vi "IMAQ FPGA Camera Link Overflow Check.vi"(9 "Max Index":u16, 10 "Read Info":T2, 11 "Write Info":T3) -> (3 "Overlfow":bool)   [LabVIEW 2017]
uses:
  <vilib>/visionFPGA/Basics/Camera Link Acquisition/Controls/IMAQ FPGA Camera Link Line Builder State.ctl
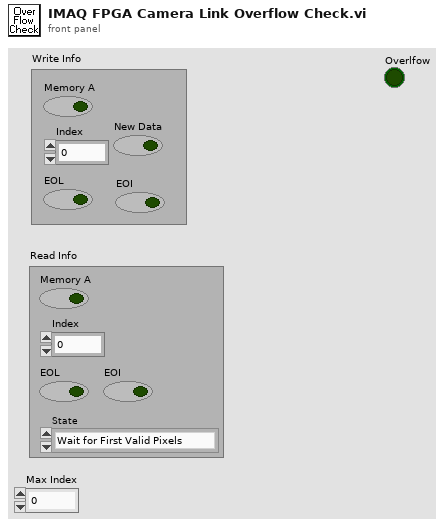
[diagram p1: front panel]
types:
  T1 = typedef "IMAQ FPGA Camera Link Line Builder State.ctl" = enum16{"Wait for First Valid Pixels", "Update Section 1", "Update Section 2", "Update Section 3", "Update Last Section", "Add Final Pack", "Add End of Line", "Check End of Image"}
  T2 = cluster{"Memory A":bool, "Index":u16, "EOL":bool, "State":T1, "EOI":bool}
  T3 = cluster{"Memory A":bool, "Index":u16, "EOL":bool, "New Data":bool, "EOI":bool}
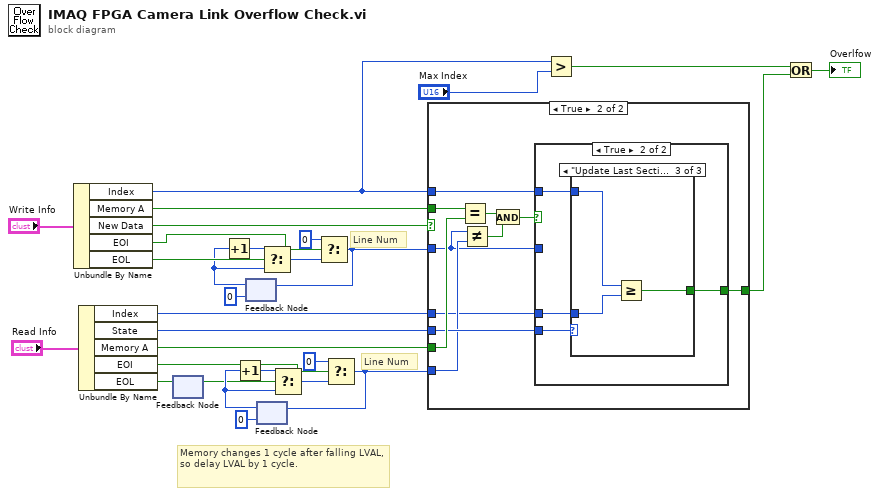
[diagram p0: block diagram]
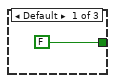
[diagram p4: hidden frame]
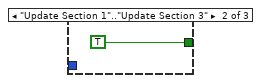
[diagram p5: hidden frame]
diagram:
  # "Line Num"
  # "Line Num"
  # "Memory changes 1 cycle after falling LVAL, so delay LVAL by 1 cycle."
  n1 = Unbundle By Name("Write Info") -> ("Index"=w7:u16, "Memory A"=w12:bool, "New Data"=w20:bool, "EOI"=w24:bool, "EOL"=w28:bool)
  n2 = Unbundle By Name("Read Info") -> ("Index"=w9:u16, "State"=w10:T1, "Memory A"=w11:bool, "EOI"=w13:bool, "EOL"=w14:bool)
  n3 = feedback-in #1(w14) -> ()
  n4 = feedback #1() -> (w8:bool)  [unwired: 1 in]
  n5 = feedback #2(u16 0) -> (w25:u16)
  n6 = Increment(x=w25) -> (x+1=w26:u16)
  n7 = feedback #3(u16 0) -> (w17:u16)
  n8 = Increment(x=w17) -> (x+1=w16:u16)
  n9 = Select(t=w26, s=w28, f=w25) -> (s? t:f=w23:u16)
  n10 = Select(t=w16, s=w8, f=w17) -> (s? t:f=w18:u16)
  n11 = Select(t=u16 0, s=w24, f=w23) -> (s? t:f=w2:u16)
  n12 = feedback-in #2(w2) -> ()
  n13 = Select(t=u16 0, s=w13, f=w18) -> (s? t:f=w1:u16)
  n14 = feedback-in #3(w1) -> ()
  n15 = case shown="True" w20 {
    tunnel: w1 -> [_ w36]
    tunnel: w2 -> [_ w33]
    tunnel: w12 -> [_ w40]
    tunnel: w11 -> [_ w39]
    tunnel: w10 -> [_ w38]
    tunnel: w7 -> [_ w30]
    tunnel: w9 -> [_ w32]
    tunnel: [_ w31] -> w4
    frame False {
    }
    frame True {
      n16 = Equal?(x=w40, y=w39) -> (x = y?=w37:bool)
      n17 = Not Equal?(x=w33, y=w36) -> (x != y?=w35:bool)
      n18 = And(x=w37, y=w35) -> (x .and. y?=w34:bool)
      n19 = case shown="True" w34 {
        tunnel: w38 -> [_ w44]
        tunnel: w33 -> [_ _]
        tunnel: w32 -> [_ w41]
        tunnel: [_ w43] -> w31
        tunnel: w30 -> [_ w42]
        frame False {
        }
        frame True {
          n20 = case shown="\"Update Last Section\"" w44 {
            tunnel: [FALSE TRUE w47] -> w43
            tunnel: w42 -> [_ _ w49]
            tunnel: w41 -> [_ _ w48]
            frame Default {
            }
            frame "Update Section 1".."Update Section 3" {
            }
            frame "Update Last Section" {
              n21 = Greater Or Equal?(x=w49, y=w48) -> (x >= y?=w47:bool)
            }
          }
        }
      }
    }
  }
  n22 = Greater?(x=w7, y="Max Index") -> (0:w5:bool)
  n23 = Or(x=w5, y=w4) -> (x .or. y?=→"Overlfow":bool)
